vi "Start Deploy.vi"(11 "NetCPU in":refnum<class "NetCPU.lvclass">) -> (3 "NetCPU out":refnum<class "NetCPU.lvclass">)   [LabVIEW 2020, in "NI_TargetHelper.lvlib" / "NetCPU.lvclass"]
uses:
  <vilib>/TargetSupport/NI_TargetHelper/NetCPU/NetCPU.lvclass
  <vilib>/TargetSupport/NI_TargetHelper/NetCPU/NetCPU.lvclass/NetCPU.ctl
  <vilib>/TargetSupport/NI_TargetHelper/NI_TargetHelper.lvlib
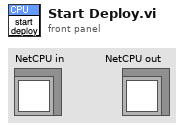
[diagram p1: front panel]
types:
  T1 = enum16{"Share clones between instances", "Preallocate clone for each instance"}
  T2 = typedef "NI_TargetHelper.lvlib/Instance VIref.ctl" = refnum<vi>
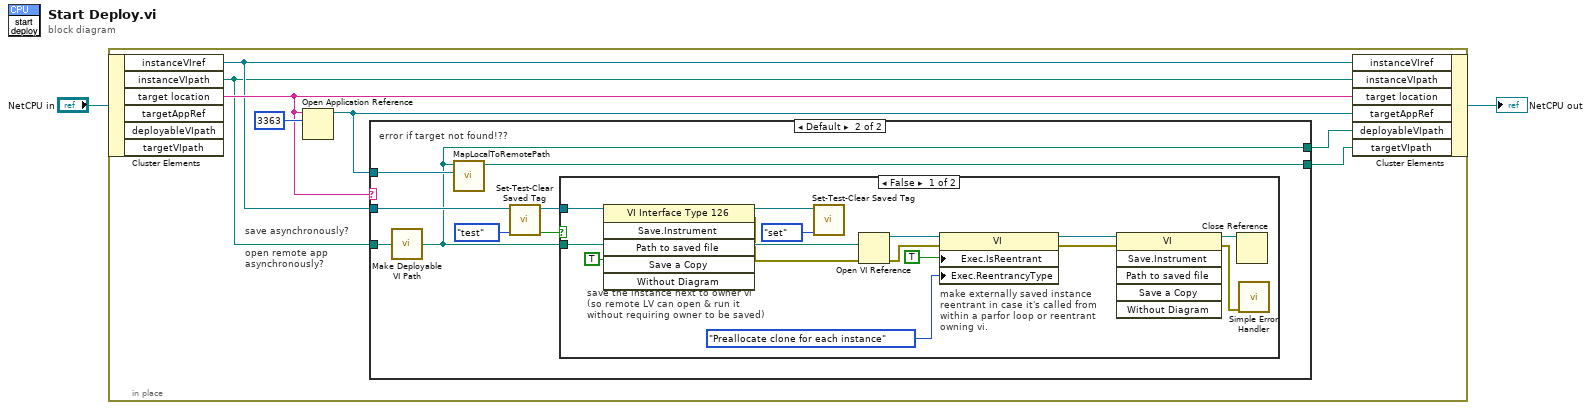
[diagram p0: block diagram]
diagram:
  n1 = in-place {
    # "save asynchronously?\n\nopen remote app \nasynchronously?"
    n2 = in-place-cluster #1("NetCPU in") -> ("instanceVIref"=w6:T2, "instanceVIpath"=w5:path, "target location"=w8:string)  [unwired: 3 out]
    n3 = Open Application Reference(10:u16 3363 ("remote port or service name"), 11:w8) -> (3:w7:refnum<vi>)  [unwired: 2 in, 1 out]
    n4 = case shown="Default" w8 {
      tunnel: w6 -> [_ w17]
      tunnel: w5 -> [_ w11]
      tunnel: [_ w13] -> w4
      tunnel: w7 -> [_ w12]
      tunnel: [_ w10] -> w3
      frame "" {
      }
      frame Default {
        # "error if target not found!??"
        n5 = call <vilib>:"Make Deployable VI Path.vi"("instance path"=w11) -> ("deployable path"=w10:path)
        n6 = call <vilib>:"MapLocalToRemotePath.vi"("appref"=w12, "local path"=w10) -> ("remote path"=w13:path)  [unwired: 9 in]
        n7 = call <vilib>:"Set-Test-Clear Saved Tag.vi"("op"=enum16{"test", "clear", "set"}."test", "instVIref"=w17) -> ("saved"=w14:bool, "instVIref out"=w16:T2)  [unwired: 8 in]
        n8 = case shown="False" w14 {
          tunnel: w16 -> [w30 _]
          tunnel: w10 -> [w25 _]
          frame False {
            # "make externally saved instance\nreentrant in case it's called from\nwithin a parfor loop or reentrant\nowning vi."
            # "save the instance next to owner vi\n(so remote LV can open & run it\nwithout requiring owner to be saved)"
            n9 = invoke class="VI Interface Type 126" method="Save.Instrument"(reference=w30, "Path to saved file"=w25, "Save a Copy"=TRUE) -> (reference out=w29:T2, error out=w19:errorcluster)  [unwired: 3 in, 4 out]
            n10 = call <vilib>:"Set-Test-Clear Saved Tag.vi"("op"=enum16{"test", "clear", "set"}."set", "instVIref"=w29) -> ()  [unwired: 8 in, 2 out]
            n11 = Open VI Reference(vi path=w25, error in (no error)=w19) -> (vi reference=w24:refnum<vi>, error out=w18:errorcluster)  [unwired: 4 in]
            n12 = property class="VI"(reference=w24, error in=w18, "Exec.IsReentrant"=TRUE ("Execution:Is Reentrant"), "Exec.ReentrancyType"=T1."Preallocate clone for each instance" ("Execution:Reentrancy Type")) -> (reference out=w23:refnum<vi>, error out=w21:errorcluster)
            n13 = invoke class="VI" method="Save.Instrument"(reference=w23, error in=w21) -> (reference out=w22:refnum<vi>, error out=w20:errorcluster)  [unwired: 4 in, 4 out]
            n14 = Close Reference(reference=w22) -> ()  [unwired: 1 in, 1 out]
            n15 = call <vilib>:"Simple Error Handler.vi"("error in (no error)"=w20) -> ()  [unwired: 4 in, 5 out]
          }
          frame True {
          }
        }
      }
    }
    n16 = in-place-cluster #1("instanceVIref"=w6, "instanceVIpath"=w5, "target location"=w8, "targetAppRef"=w7, "deployableVIpath"=w3, "targetVIpath"=w4) -> (→"NetCPU out":refnum<class "NetCPU.lvclass">)
  }
